vi "VeriStand DSF.Transfer.Configuration.Get Direction.vi"(11 "VeriStand DSF.Transfer.Configuration in":refnum<class "VeriStand DSF.Transfer.Configuration.lvclass">=refnum) -> (2 "Direction":T1, 3 "VeriStand DSF.Transfer.Configuration out":refnum<class "VeriStand DSF.Transfer.Configuration.lvclass">)   [LabVIEW 2017, in "Data Sharing Custom Device Engine.lvlib" / "VeriStand DSF.Transfer.Configuration.lvclass"]
uses:
  VeriStand DSF.Transfer.Configuration.lvclass
  Builds/Data Sharing Framework/Current/Data Sharing Framework Core/DSF Core.lvlibp/DSF Configuration API/Public/Controls/DSF Direction.ctl
  VeriStand DSF.Transfer.Configuration.lvclass/VeriStand DSF.Transfer.Configuration.ctl
  Builds/Data Sharing Framework/Current/Data Sharing Framework Core/DSF Core.lvlibp
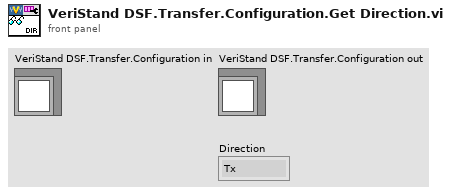
[diagram p1: front panel]
types:
  T1 = typedef "DSF Core.lvlibp/DSF Direction.ctl" = enum8{"Tx", "Rx"}
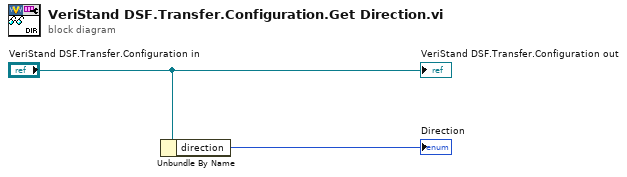
[diagram p0: block diagram]
diagram:
  n1 = Unbundle By Name("VeriStand DSF.Transfer.Configuration in") -> ("direction"=→"Direction":T1)
  "VeriStand DSF.Transfer.Configuration out" <- "VeriStand DSF.Transfer.Configuration in"
